vi "Update MemberTable In Excel.vi"(8 "error in (no error)":errorcluster, 11 "MemberTable in":refnum<class "TimeTable.lvclass">) -> (0 "error out":errorcluster, 3 "MemberTable out":refnum<class "TimeTable.lvclass">)   [LabVIEW 2015, in "TimeTable.lvclass"]
uses:
  TimeTable.lvclass
  TimeTable.lvclass/TimeTable.ctl
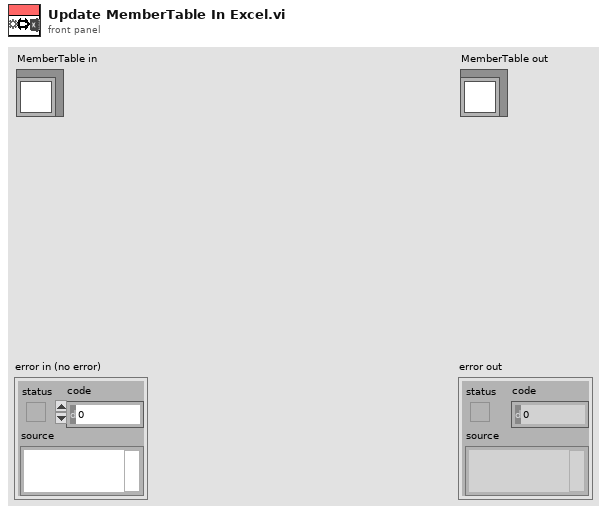
[diagram p1: front panel]
types:
  T1 = typedef "TimeTable.lvclass/Table_Cell.ctl" = cluster{"结束周":i32, "起始周":i32, "课程名称":string}
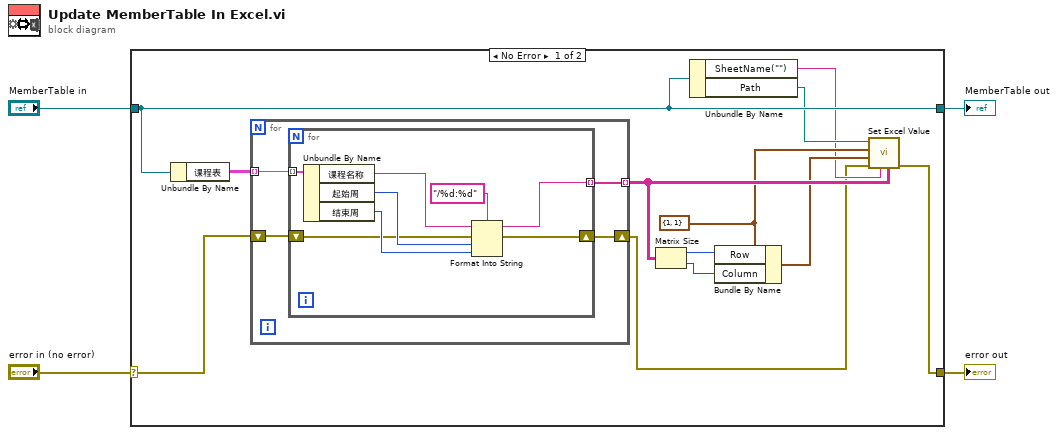
[diagram p0: block diagram]
diagram:
  n1 = case shown="No Error" "error in (no error)" {
    selector: "error in (no error)" -> [w15 w30]
    tunnel: [w5 w30] -> w3
    tunnel: [w9 w29] -> w1
    tunnel: "MemberTable in" -> [w9 w29]
    frame No Error {
      w10 = cluster{"Column":i32, "Row":i32} {"Column"=1, "Row"=1} ("Start")
      n2 = Unbundle By Name(w9) -> ("课程表"=w16:T1[][])
      n3 = for {
        tunnel: w16 -> [w20] mode=indexing
        shift-right: [w18] -> w6
        shift-left: w15 -> [w19]
        tunnel: [w17] -> w14 mode=indexing
        n4 = for {
          tunnel: w20 -> [w28] mode=indexing
          shift-right: [w22] -> w18
          shift-left: w19 -> [w23]
          tunnel: [w21] -> w17 mode=indexing
          n5 = Unbundle By Name(w28) -> ("课程名称"=w24:string, "起始周"=w27:i32, "结束周"=w25:i32)
          n6 = Format Into String(format string="/%d:%d", initial string=w24, error in=w23, w27, w25) -> (resulting string=w21:string, error out=w22:errorcluster)
        }
      }
      n7 = Matrix Size(0:w14) -> (1:w13:i32, 2:w12:i32)
      n8 = Unbundle By Name(w9) -> ("SheetName(\"\")"=w7:string, "Path"=w8:path)
      n9 = Bundle By Name(cluster=w10, "Row"=w13, "Column"=w12) -> (w11:cluster{"Column":i32, "Row":i32})
      n10 = call "Set Excel Value.vi"("Excel_Values"=w14, "SheetName(\"\")"=w7, "error in (no error)"=w6, "End"=w11, "Start"=w10, "path"=w8) -> ("error out"=w5:errorcluster)  [unwired: 5 in]
    }
    frame Error {
    }
  }
  "error out" <- w3
  "MemberTable out" <- w1
